vi "Dequeue Master and Local.vi"(8 "error in (no error)":errorcluster, 10 "Master":refnum<queue>, 11 "UI":refnum<queue>) -> (0 "error out":errorcluster, 1 "Message Data":variant, 2 "Message":string, 3 "UI out":refnum<queue>)   [LabVIEW 2013, in "AvaSpec.lvlib" / "AvaSpec Message Queue.lvlib"]
uses:
  AvaSpec Message Queue.lvlib
  Message Cluster.ctl
  Settings/Settings.ctl
  Acquisition/Hardware Configuration.ctl
  Libraries/AS-5216-DLL/AVS settings.ctl
  Acquisition/Sphere Indicator.ctl
  Settings/Measurement Type.ctl
  Logging/Logging Configuration.ctl
  AvaSpec.lvlib
  Acquisition/AvaSpec Acquisition.lvlib
  Logging/AvaSpec Logging.lvlib
  Settings/AvaSpec Settings.lvlib
panel:
  in  "Settings":T1
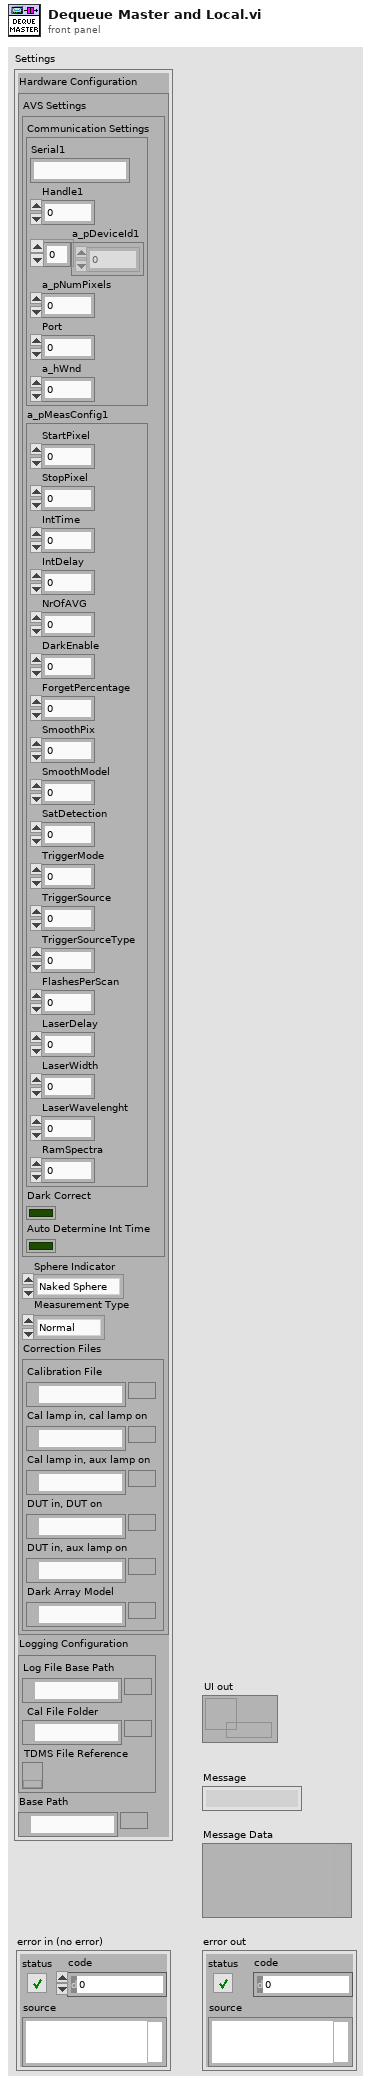
[diagram p1: front panel]
types:
  T1 = typedef "AvaSpec.lvlib/AvaSpec Settings.lvlib/Settings.ctl" = cluster{"Hardware Configuration":T2, "Logging Configuration":T6, "Base Path":path}
  T2 = typedef "AvaSpec.lvlib/AvaSpec Acquisition.lvlib/Hardware Configuration.ctl" = cluster{"AVS Settings":T3, "Sphere Indicator":T4, "Measurement Type":T5, "Correction Files":cluster{"Calibration File":path, "Cal lamp in, cal lamp on":path, "Cal lamp in, aux lamp on":path, "DUT in, DUT on":path, "DUT in, aux lamp on":path, "Dark Array Model":path}}
  T3 = typedef "AvaSpec.lvlib/AVS settings.ctl" = cluster{"Communication Settings":cluster{"Serial1":string, "Handle1":i32, "a_pDeviceId1":u8[], "a_pNumPixels":u16, "Port":i32, "a_hWnd":i32}, "a_pMeasConfig1":cluster{"StartPixel":u16, "StopPixel":u16, "IntTime":sgl, "IntDelay":u32, "NrOfAVG":u32, "DarkEnable":u8, "ForgetPercentage":u8, "SmoothPix":u16, "SmoothModel":u8, "SatDetection":u8, "TriggerMode":u8, "TriggerSource":u8, "TriggerSourceType":u8, "FlashesPerScan":u16, "LaserDelay":u32, "LaserWidth":u32, "LaserWavelenght":sgl, "RamSpectra":u16}, "Dark Correct":bool, "Auto Determine Int Time":bool}
  T4 = typedef "AvaSpec.lvlib/Sphere Indicator.ctl" = enum16{"Naked Sphere", "Insulated Sphere"}
  T5 = typedef "Measurement Type.ctl" = enum16{"Normal", "Calibration", "Dark"}
  T6 = typedef "AvaSpec.lvlib/AvaSpec Logging.lvlib/Logging Configuration.ctl" = cluster{"Log File Base Path":path, "Cal File Folder":path, "TDMS File Reference":refnum<k34>}
  T7 = typedef "AvaSpec.lvlib/AvaSpec Message Queue.lvlib/Message Cluster.ctl" = cluster{"Message":string, "Message Data":variant}
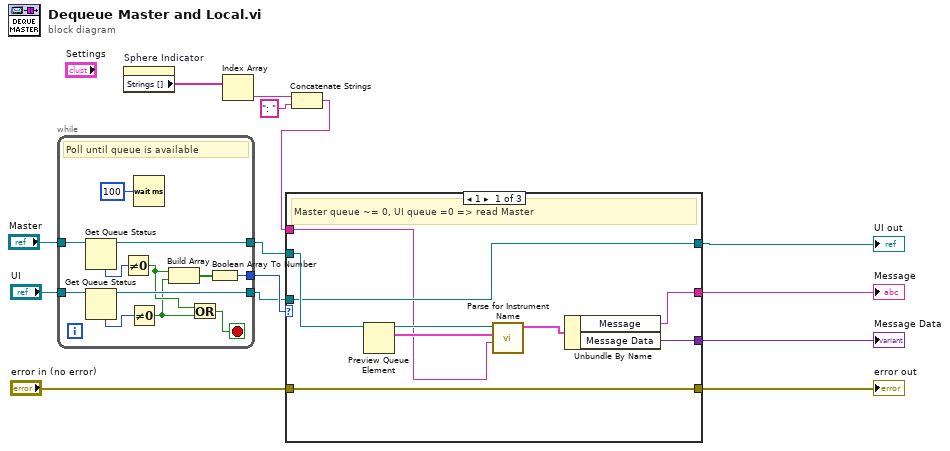
[diagram p0: block diagram]
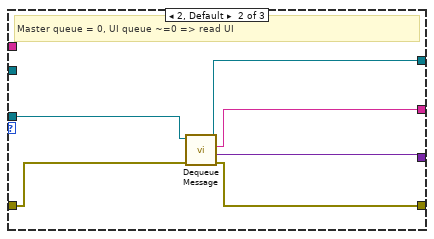
[diagram p2: hidden frame]
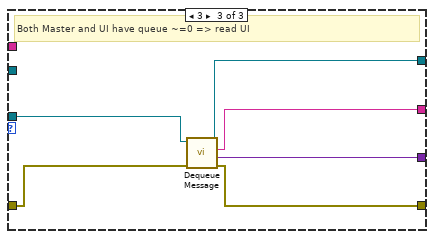
[diagram p3: hidden frame]
diagram:
  n1 = while {
    tunnel: "UI" -> [w26]
    tunnel: "Master" -> [w23]
    tunnel: [w21] -> w12
    tunnel: [w20] -> w11
    tunnel: [w19] -> w10
    stop <- w17 stop-if-true
    # "Poll until queue is available"
    n2 = Get Queue Status(queue=w23) -> (queue out=w20:refnum<queue>, # elements in queue=w24:i32)  [unwired: 2 in, 6 out]
    n3 = Get Queue Status(queue=w26) -> (queue out=w19:refnum<queue>, # elements in queue=w25:i32)  [unwired: 2 in, 6 out]
    n4 = Not Equal To 0?(x=w24) -> (x != 0?=w16:bool)
    n5 = Not Equal To 0?(x=w25) -> (x != 0?=w15:bool)
    n6 = Wait (ms)(milliseconds to wait=u32 100) -> ()  [unwired: 1 out]
    n7 = Build Array(w16, w15) -> (w22:bool[])
    n8 = Or(x=w16, y=w15) -> (x .or. y?=w17:bool)
    n9 = Boolean Array To Number(Boolean array=w22) -> (number=w21:u32)
  }
  n10 = property on="Sphere Indicator" class="Enum (strict)"() -> ("Strings []"=w2:string[])  [unwired: 2 in, 2 out]
  n11 = Index Array(array=w2) -> (element=w3:string)  [unwired: 1 in]
  n12 = Concatenate Strings(w3, ": " ("string")) -> (w1:string)
  n13 = case shown="1" w12 {
    tunnel: w11 -> [w32 _ _]
    tunnel: w10 -> [w28 w37 w42]
    tunnel: "error in (no error)" -> [w33 w38 w47]
    tunnel: [w28 w36 w43] -> w8
    tunnel: [w35 w41 w44] -> w7
    tunnel: [w34 w40 w45] -> w6
    tunnel: [w33 w39 w46] -> w5
    tunnel: w1 -> [w27 _ _]
    frame 1 {
      # "Master queue ~= 0, UI queue =0 => read Master"
      n14 = Preview Queue Element(queue=w32) -> (queue out=w31:refnum<queue>, element=w30:T7)  [unwired: 2 in, 2 out]
      n15 = call "Parse for Instrument Name.vi"("Instrument Name"=w27, "Message In"=w30, "Message Queue"=w31) -> ("Message Out"=w29:T7)  [unwired: 8 in]
      n16 = Unbundle By Name(w29) -> ("Message"=w35:string, "Message Data"=w34:variant)
    }
    frame 2, Default {
      # "Master queue = 0, UI queue ~=0 => read UI"
      n17 = call "Dequeue Message.vi"("error in (no error)"=w38, "Message Queue"=w37) -> ("error out"=w39:errorcluster, "Message Data"=w40:variant, "Message"=w41:string, "dup Message Queue"=w36:refnum<queue>)  [unwired: 6 in]
    }
    frame 3 {
      # "Both Master and UI have queue ~=0 => read UI"
      n18 = call "Dequeue Message.vi"("error in (no error)"=w47, "Message Queue"=w42) -> ("error out"=w46:errorcluster, "Message Data"=w45:variant, "Message"=w44:string, "dup Message Queue"=w43:refnum<queue>)  [unwired: 6 in]
    }
  }
  "error out" <- w5
  "Message Data" <- w6
  "Message" <- w7
  "UI out" <- w8
